vi "PH_Beckhoff.scale digital DIM Value.vi"(0 "DIM value":bool, 1 "inverted?":bool) -> (2 "Beckhoff value":bool)   [LabVIEW 2014, in "PH_Beckhoff.lvlib"]
doc: "This VI is forseen to scale (this means: invert) the DIM value to the raw digital Beckhoff value to be set."
uses:
  PH_Beckhoff.lvlib
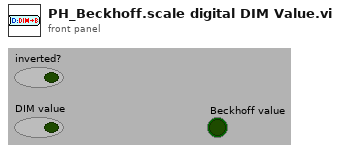
[diagram p1: front panel]
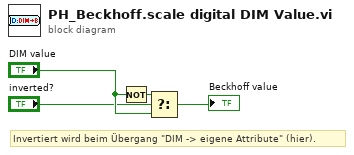
[diagram p0: block diagram]
diagram:
  # "Invertiert wird beim Übergang \"DIM -> eigene Attribute\" (hier)."
  n1 = Not(x="DIM value") -> (.not. x?=w3:bool)
  n2 = Select(t=w3, s="inverted?", f="DIM value") -> (s? t:f=→"Beckhoff value":bool)
